vi "CMN_CheckDisk.vi"(6 "DHE_DBSRef":T1, 7 "num_images (1)":i32=1, 8 "error in":errorcluster, 9 "Generate Error?":bool, 10 "size in":dbl format="%.2f", 11 "path":path) -> (0 "error out":errorcluster, 2 "free disk":dbl format="%.2f", 3 "total Size":dbl format="%.2f")   [LabVIEW 2016]
uses:
  DBSHAND/private/vis/DatabaseHand_RefNum.ctl
  DBSHAND/private/vis/DatabaseHand_Element_Get(bool).vi
panel:
  in  "create?":bool
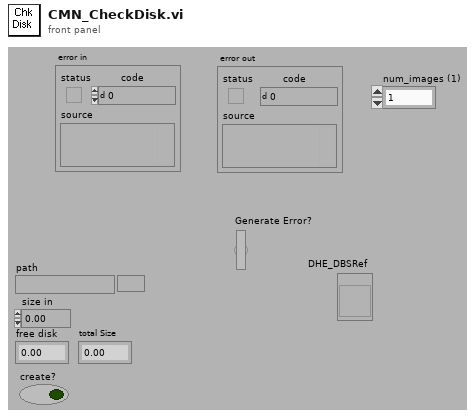
[diagram p1: front panel]
types:
  T1 = typedef "DatabaseHand_RefNum.ctl" = refnum<vi>
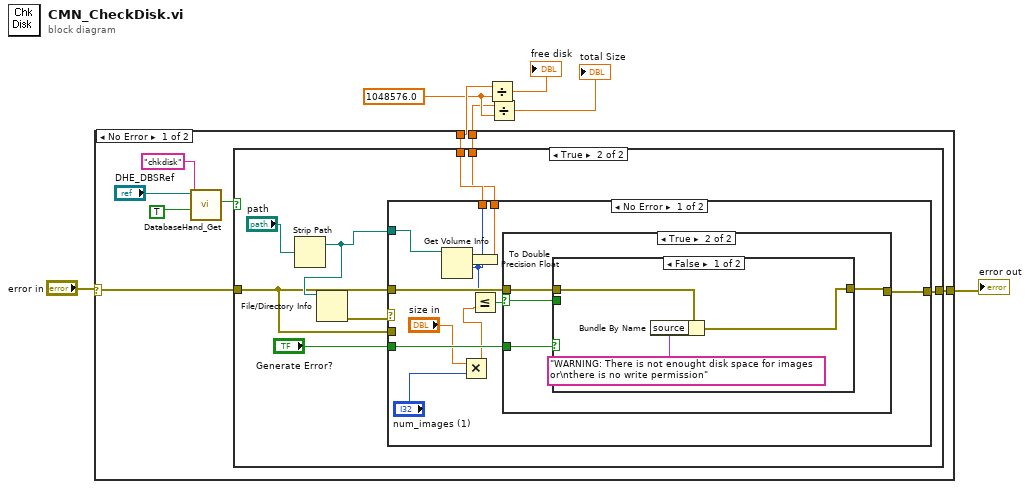
[diagram p0: block diagram]
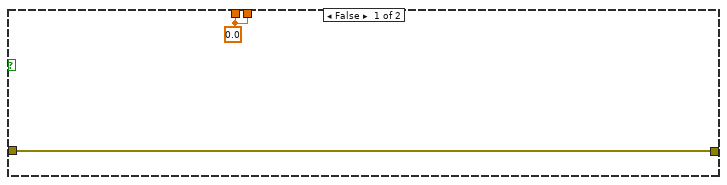
[diagram p2: hidden frame]
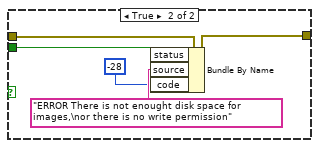
[diagram p4: hidden frame]
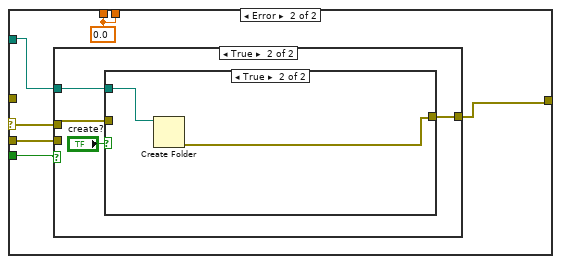
[diagram p5: hidden frame]
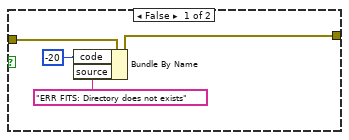
[diagram p7: hidden frame]
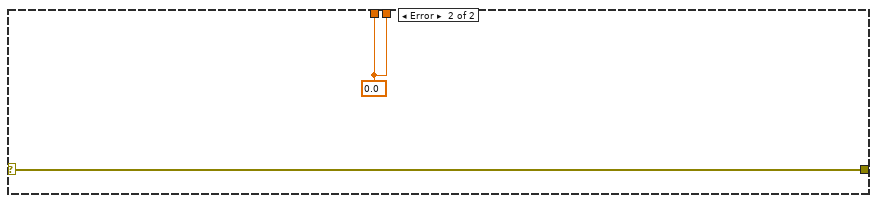
[diagram p8: hidden frame]
diagram:
  w3 = 1048576.0 ("y")
  n1 = case shown="No Error" "error in" {
    selector: "error in" -> [w12 w68]
    tunnel: [w15 w68] -> w7
    tunnel: [w14 w67] -> w4
    tunnel: [w13 w67] -> w2
    frame No Error {
      n2 = call-poly "DatabaseHand_Get.vi"("default value"=TRUE, "name"="chkdisk", "Database RefNum in"="DHE_DBSRef") -> ("value"=w8:bool)  [unwired: 2 in, 6 out]
      n3 = case shown="True" w8 {
        tunnel: [w16 w25] -> w15
        tunnel: [w17 w24] -> w14
        tunnel: [w17 w23] -> w13
        tunnel: w12 -> [w16 w18]
        frame False {
          w17 = 0.0 ("free")
        }
        frame True {
          n4 = Strip Path(path="path") -> (stripped path=w20:path)  [unwired: 1 out]
          n5 = File/Directory Info(path=w20) -> (error out=w22:errorcluster)  [unwired: 1 in, 6 out]
          n6 = case shown="No Error" w22 {
            selector: w22 -> [_ w54]
            tunnel: [w35 w53] -> w25
            tunnel: w18 -> [w34 _]
            tunnel: [w33 w55] -> w24
            tunnel: [w32 w55] -> w23
            tunnel: w20 -> [w31 w52]
            tunnel: "Generate Error?" -> [w30 w51]
            tunnel: w18 -> [_ w50]
            frame No Error {
              n7 = Get Volume Info(11:w31) -> (1:w33:i64, 2:w26:i64)  [unwired: 1 in, 4 out]
              n8 = Multiply(x="size in", y="num_images (1)") -> (x*y=w27:dbl)
              n9 = To Double Precision Float(number=w26) -> (double precision float=w32:dbl)
              n10 = Less Or Equal?(x=w33, y=w27) -> (x <= y?=w36:bool)
              n11 = case shown="True" w36 {
                selector: w36 -> [_ w39]
                tunnel: w34 -> [w37 w41]
                tunnel: [w37 w40] -> w35
                tunnel: w30 -> [_ w38]
                frame False {
                }
                frame True {
                  n12 = case shown="False" w38 {
                    tunnel: w41 -> [w44 w49]
                    tunnel: [w43 w48] -> w40
                    tunnel: w39 -> [_ w47]
                    frame False {
                      n13 = Bundle By Name(cluster=w44, "source"="WARNING: There is not enought disk space for images or\nthere is no write permission") -> (w43:errorcluster)
                    }
                    frame True {
                      n14 = Bundle By Name(cluster=w49, "status"=w47, "source"="ERROR There is not enought disk space for images,\nor there is no write permission", "code"=-28) -> (w48:errorcluster)
                    }
                  }
                }
              }
            }
            frame Error {
              w55 = 0.0 ("free")
              n15 = case shown="True" w51 {
                tunnel: w54 -> [_ w60]
                tunnel: [w56 w59] -> w53
                tunnel: w52 -> [_ w57]
                tunnel: w50 -> [w56 _]
                frame False {
                }
                frame True {
                  n16 = case shown="True" "create?" {
                    tunnel: w60 -> [w64 _]
                    tunnel: [w63 w65] -> w59
                    tunnel: w57 -> [_ w66]
                    frame False {
                      n17 = Bundle By Name(cluster=w64, "code"=-20, "source"="ERR FITS: Directory does not exists") -> (w63:errorcluster)
                    }
                    frame True {
                      n18 = Create Folder(path (use dialog)=w66) -> (error out=w65:errorcluster)  [unwired: 1 in, 3 out]
                    }
                  }
                }
              }
            }
          }
        }
      }
    }
    frame Error {
      w67 = 0.0 ("free")
    }
  }
  "error out" <- w7
  n19 = Divide(x=w4, y=w3) -> (x/y=→"free disk":dbl)
  n20 = Divide(x=w2, y=w3) -> (x/y=→"total Size":dbl)
